vi "超标留样启动命令.vi"   [LabVIEW 2016]
uses:
  DR803M4/DR803M4.lvlib
types:
  T1 = enum16{"德润DR803M", "德润DR803L", "德润DR803F", "科盛超标留样", "德润DR803M4"}
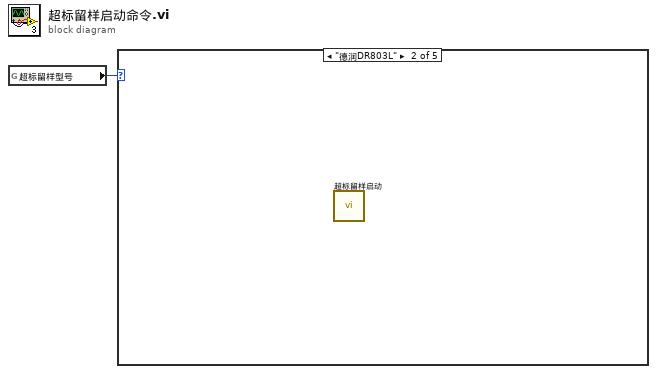
[diagram p0: block diagram]
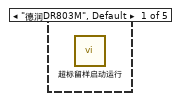
[diagram p2: hidden frame]
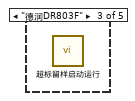
[diagram p3: hidden frame]
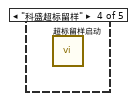
[diagram p4: hidden frame]
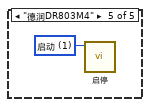
[diagram p5: hidden frame]
diagram:
  n1 = global read "断电保存全局.vi" "超标留样型号"() -> (w1:T1)
  n2 = case shown="\"德润DR803L\"" w1 {
    frame "德润DR803M", Default {
      n3 = call "超标留样启动运行.vi"() -> ()  [unwired: 11 in, 1 out]
    }
    frame "德润DR803L" {
      n4 = call "超标留样启动.vi"() -> ()  [unwired: 11 in, 1 out]
    }
    frame "德润DR803F" {
      n5 = call "超标留样启动运行.vi"() -> ()  [unwired: 11 in, 1 out]
    }
    frame "科盛超标留样" {
      n6 = call "超标留样启动.vi"() -> ()  [unwired: 11 in, 1 out]
    }
    frame "德润DR803M4" {
      w2 = u16 1 items=["停止", "启动"] ("启停")
      n7 = call "启停.vi"("启停"=w2) -> ()  [unwired: 10 in, 1 out]
    }
  }
